vi "Transfer Data to Host DMA.vi"(11 "Settings.DMA":cluster{"# of Injectors":u8}={"# of Injectors"=6}) -> (2 "Intermediate Time Out?":bool, 3 "Host DMA Out?":bool)   [LabVIEW 2015]
uses:
  <vilib>/rvi/DataTransferAndStorage/Container/Common/niFpgaContainerExecOnDevCompGetState.vi
  <vilib>/rvi/Emulation/niFpgaEmulationIsFPGAContextNoSignature.vi
  <vilib>/rvi/Emulation/niFpgaSctlEmulationGetInTimedLoop.vi
  <vilib>/rvi/errors/niFpgaSetErrorForExecOnDevCompSimple.vi
  <vilib>/rvi/eio/common/nirviEmuReportErrorAndStop.vi
  <vilib>/rvi/DataTransferAndStorage/Container/Common/niFpgaContainerGetUniqueNameForEmu.vi
  <vilib>/rvi/FIFO/Fifo_Resource/nirvififoEmulationSetSize.vi
  <vilib>/rvi/FIFO/Fifo_Resource/nirviFifoEmulationQueueMgr.vi
  <instcachedir>/0/nirviFifoEmulationQueueMgr_E5CAEC123FF24DC58D834DCA3CDAA9B5.lvgen/nirviFifoEmulationQueueMgr_E5CAEC123FF24DC58D834DCA3CDAA9B5_001.vi
  <vilib>/rvi/FIFO/Fifo_Resource/nirvififoEmulationDetermineInputValidOut.vi
  <vilib>/rvi/FIFO/Fifo_Resource/nirvififoEmulationCreateLock.vi
  <vilib>/rvi/Emulation/niFpgaProcessEmulError.vi
  <vilib>/rvi/FIFO/Fifo_Resource/nirvififoEmulationObtainLock.vi
  <vilib>/rvi/FIFO/Fifo_Resource/nirvififoEmulationReleaseLock.vi
  <vilib>/rvi/occurrence/nirviWaitOnOccurrenceBase.vi
  <vilib>/rvi/errors/nirviReportUnexpectedCaseInternalError.vi
  <vilib>/rvi/errors/nirviReportUnexpectedCaseInternalError (U32).vi
  <vilib>/Utility/error.llb/Clear Errors.vi
  <vilib>/rvi/interface/RandomDataEmulation/niFpgaRandomDataHandleErrors.vi
  <instcachedir>/0/nirviFifoEmulationQueueMgr_E5CAEC123FF24DC58D834DCA3CDAA9B5.lvgen/nirviFifoEmulationQueueMgr_E5CAEC123FF24DC58D834DCA3CDAA9B5_008.vi
  <vilib>/rvi/DataTransferAndStorage/Container/XNode/niFpgaContainer.xnode
  <vilib>/rvi/FIFO/Fifo_Resource/niFpgaFifoEmulationRefIn.vi
  <vilib>/rvi/interface/RandomDataEmulation/nirviRandomDataFpgaReadWriteTemplate.vi
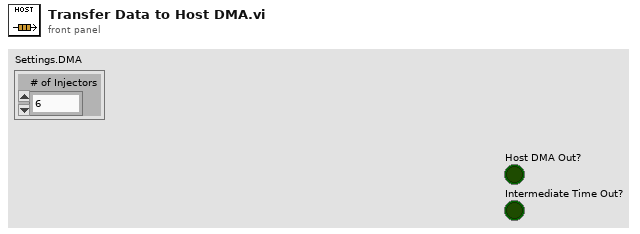
[diagram p1: front panel]
types:
  T1 = cluster{"# of samples captured":u16, "# Transition Elements":u16, "Injector Index":u8, "Iteration":u32}
  T2 = enum8{"Wait on Transfer", "Transfer Injector Index", "Transfer # of Samples", "Transfer # of Transitions", "Transfer Transitions", "Transfer Voltage Samples", "Transfer Current Samples"}
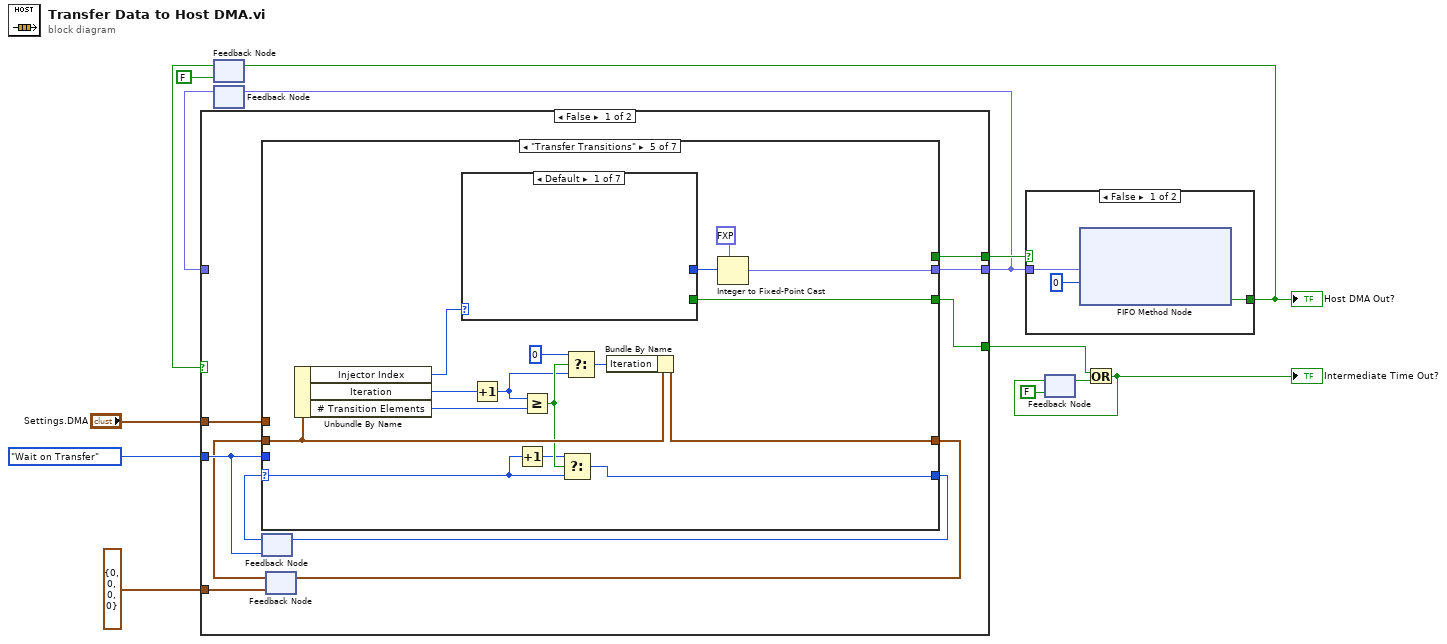
[diagram p0: block diagram]
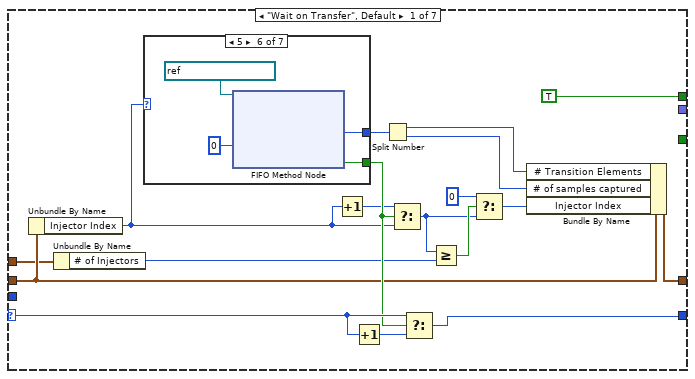
[diagram p2: hidden frame]
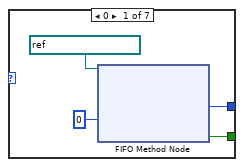
[diagram p3: hidden frame]
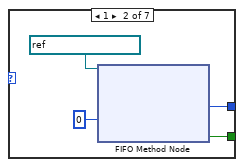
[diagram p4: hidden frame]
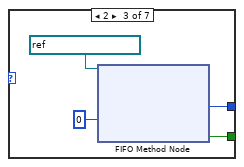
[diagram p5: hidden frame]
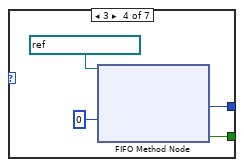
[diagram p6: hidden frame]
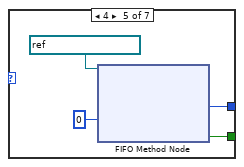
[diagram p7: hidden frame]
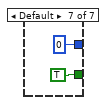
[diagram p8: hidden frame]
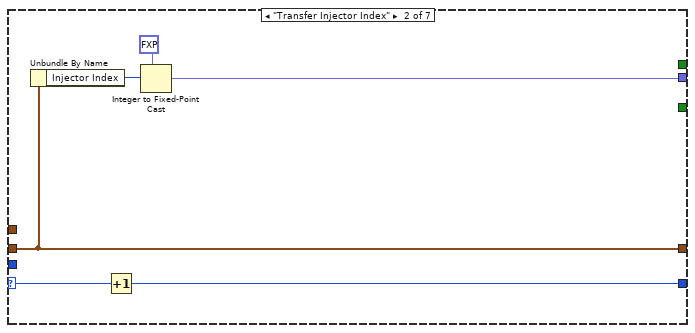
[diagram p9: hidden frame]
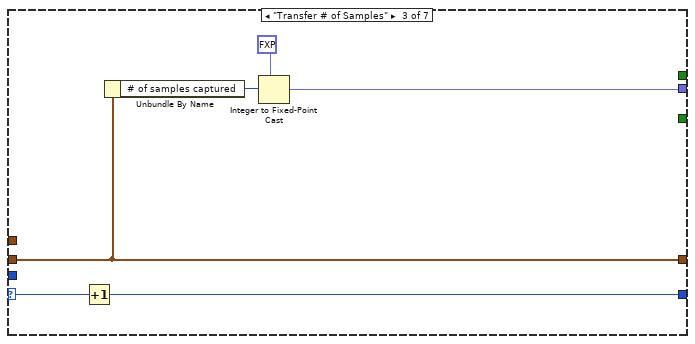
[diagram p10: hidden frame]
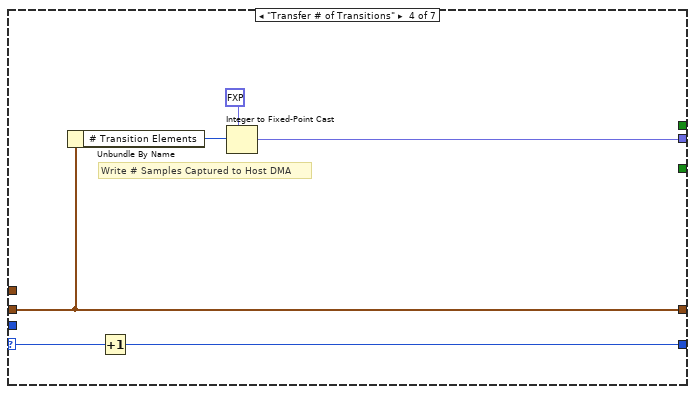
[diagram p11: hidden frame]
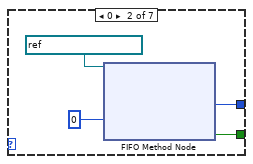
[diagram p12: hidden frame]
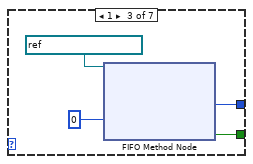
[diagram p13: hidden frame]
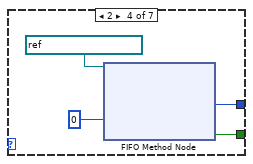
[diagram p14: hidden frame]
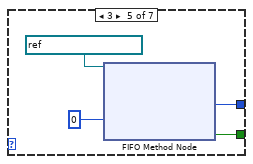
[diagram p15: hidden frame]
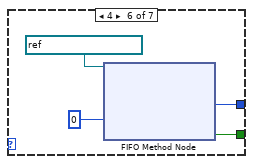
[diagram p16: hidden frame]
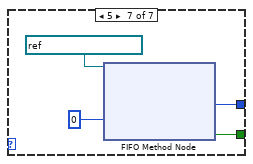
[diagram p17: hidden frame]
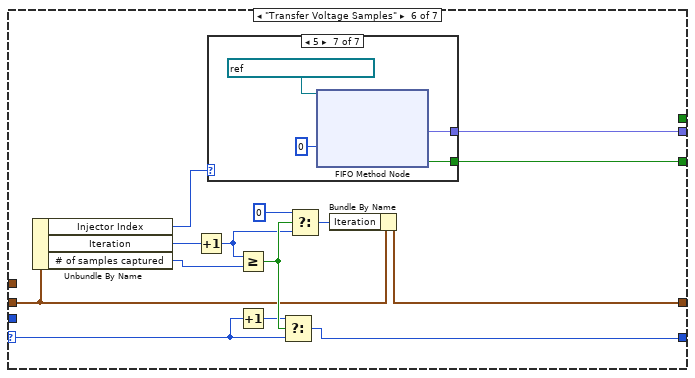
[diagram p18: hidden frame]
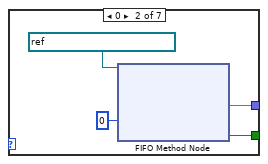
[diagram p20: hidden frame]
diagram:
  n1 = feedback #1(FALSE ("Timed Out?")) -> (w8:bool)
  n2 = feedback #2() -> (w5:fxp<+/-,32,8>)  [unwired: 1 in]
  n3 = case shown="False" w8 {
    tunnel: [w23 w203] -> w6
    tunnel: [w22 w202] -> w10
    tunnel: T2."Wait on Transfer" -> [w19 _]
    tunnel: [w18 w202] -> w1
    tunnel: "Settings.DMA" -> [w17 _]
    tunnel: T1 {"# of samples captured"=0, "# Transition Elements"=0, "Injector Index"=0, "Iteration"=0} ("Local.Data") -> [w14 _]
    tunnel: w5 -> [_ w203]
    frame False {
      n4 = feedback #3(w19) -> (w20:T2)
      n5 = feedback #4(w14) -> (w15:T1)
      n6 = case shown="\"Transfer Transitions\"" w20 {
        selector: w20 -> [w39 w73 w77 w83 w92 w132 w170]
        tunnel: w15 -> [w28 w70 w75 w80 w99 w130 w169]
        tunnel: [w37 w70 w75 w80 w100 w129 w167] -> w16
        tunnel: [w36 w72 w76 w82 w91 w131 w166] -> w21
        tunnel: [_ w69 w74 w81 w87 w128 w177] -> w23
        tunnel: [TRUE _ _ _ _ _ _] -> w22
        tunnel: w19 -> [_ _ _ _ _ _ w165]
        tunnel: [_ _ _ _ w86 w126 w164] -> w18
        tunnel: w17 -> [w25 _ _ _ _ _ _]
        frame "Wait on Transfer", Default {
          n7 = Unbundle By Name(w28) -> ("Injector Index"=w27:u8)
          n8 = Unbundle By Name(w25) -> ("# of Injectors"=w24:u8)
          n9 = case shown="5" w27 {
            tunnel: [w44 w48 w52 w56 w60 w64 u32 0 ("Element")] -> w41
            tunnel: [w43 w47 w51 w55 w59 w63 TRUE ("Timed Out?")] -> w33
            frame 0 {
              n10 = xnode ("FIFO Method Node")("Timeout"=0, "FIFO In"=refnum<k21> "Event Capture 0") -> ("Element"=w44:u32, "Timed Out?"=w43:bool)  [unwired: 1 out]
            }
            frame 1 {
              n11 = xnode ("FIFO Method Node")("Timeout"=0, "FIFO In"=refnum<k21> "Event Capture 1") -> ("Element"=w48:u32, "Timed Out?"=w47:bool)  [unwired: 1 out]
            }
            frame 2 {
              n12 = xnode ("FIFO Method Node")("Timeout"=0, "FIFO In"=refnum<k21> "Event Capture 2") -> ("Element"=w52:u32, "Timed Out?"=w51:bool)  [unwired: 1 out]
            }
            frame 3 {
              n13 = xnode ("FIFO Method Node")("Timeout"=0, "FIFO In"=refnum<k21> "Event Capture 3") -> ("Element"=w56:u32, "Timed Out?"=w55:bool)  [unwired: 1 out]
            }
            frame 4 {
              n14 = xnode ("FIFO Method Node")("Timeout"=0, "FIFO In"=refnum<k21> "Event Capture 4") -> ("Element"=w60:u32, "Timed Out?"=w59:bool)  [unwired: 1 out]
            }
            frame 5 {
              n15 = xnode ("FIFO Method Node")("Timeout"=0, "FIFO In"=refnum<k21> "Event Capture 5") -> ("Element"=w64:u32, "Timed Out?"=w63:bool)  [unwired: 1 out]
            }
            frame Default {
            }
          }
          n16 = Increment(x=w27) -> (x+1=w32:u8)
          n17 = Increment(x=w39) -> (x+1=w40:T2)
          n18 = Split Number(x=w41) -> (hi(x)=w34:u16, lo(x)=w38:u16)
          n19 = Select(t=w32, s=w33, f=w27) -> (s? t:f=w30:u8)
          n20 = Select(t=w39, s=w33, f=w40) -> (s? t:f=w36:T2)
          n21 = Greater Or Equal?(x=w30, y=w24) -> (x >= y?=w31:bool)
          n22 = Select(t=u8 0, s=w31, f=w30) -> (s? t:f=w26:u8)
          n23 = Bundle By Name(cluster=w28, "# Transition Elements"=w34, "# of samples captured"=w38, "Injector Index"=w26) -> (w37:T1)
        }
        frame "Transfer Injector Index" {
          n24 = Unbundle By Name(w70) -> ("Injector Index"=w71:u8)
          n25 = Increment(x=w73) -> (x+1=w72:T2)
          n26 = Integer to Fixed-Point Cast(fixed-point type=fxp<+/-,32,8> 0.0, integer=w71) -> (fixed-point=w69:fxp<+/-,32,8>)
        }
        frame "Transfer # of Samples" {
          n27 = Increment(x=w77) -> (x+1=w76:T2)
          n28 = Unbundle By Name(w75) -> ("# of samples captured"=w78:u16)
          n29 = Integer to Fixed-Point Cast(fixed-point type=fxp<+/-,32,8> 0.0, integer=w78) -> (fixed-point=w74:fxp<+/-,32,8>)
        }
        frame "Transfer # of Transitions" {
          # "Write # Samples Captured to Host DMA"
          n30 = Unbundle By Name(w80) -> ("# Transition Elements"=w84:u16)
          n31 = Increment(x=w83) -> (x+1=w82:T2)
          n32 = Integer to Fixed-Point Cast(fixed-point type=fxp<+/-,32,8> 0.0, integer=w84) -> (fixed-point=w81:fxp<+/-,32,8>)
        }
        frame "Transfer Transitions" {
          n33 = Unbundle By Name(w99) -> ("Injector Index"=w101:u8, "Iteration"=w95:u32, "# Transition Elements"=w96:u16)
          n34 = case shown="Default" w101 {
            tunnel: [_ w105 w109 w113 w117 w121 w125] -> w97
            tunnel: [_ w103 w107 w111 w115 w119 w123] -> w86
            frame Default {
            }
            frame 0 {
              n35 = xnode ("FIFO Method Node")("Timeout"=0, "FIFO In"=refnum<k21> "Transition FIFO 0" ("Transition FIFO")) -> ("Element"=w105:u32, "Timed Out?"=w103:bool)  [unwired: 1 out]
            }
            frame 1 {
              n36 = xnode ("FIFO Method Node")("Timeout"=0, "FIFO In"=refnum<k21> "Transition FIFO 1" ("Transition FIFO")) -> ("Element"=w109:u32, "Timed Out?"=w107:bool)  [unwired: 1 out]
            }
            frame 2 {
              n37 = xnode ("FIFO Method Node")("Timeout"=0, "FIFO In"=refnum<k21> "Transition FIFO 2" ("Transition FIFO")) -> ("Element"=w113:u32, "Timed Out?"=w111:bool)  [unwired: 1 out]
            }
            frame 3 {
              n38 = xnode ("FIFO Method Node")("Timeout"=0, "FIFO In"=refnum<k21> "Transition FIFO 3" ("Transition FIFO")) -> ("Element"=w117:u32, "Timed Out?"=w115:bool)  [unwired: 1 out]
            }
            frame 4 {
              n39 = xnode ("FIFO Method Node")("Timeout"=0, "FIFO In"=refnum<k21> "Transition FIFO 4" ("Transition FIFO")) -> ("Element"=w121:u32, "Timed Out?"=w119:bool)  [unwired: 1 out]
            }
            frame 5 {
              n40 = xnode ("FIFO Method Node")("Timeout"=0, "FIFO In"=refnum<k21> "Transition FIFO 5" ("Transition FIFO")) -> ("Element"=w125:u32, "Timed Out?"=w123:bool)  [unwired: 1 out]
            }
          }
          n41 = Increment(x=w95) -> (x+1=w89:u32)
          n42 = Increment(x=w92) -> (x+1=w93:T2)
          n43 = Greater Or Equal?(x=w89, y=w96) -> (x >= y?=w94:bool)
          n44 = Select(t=w93, s=w94, f=w92) -> (s? t:f=w91:T2)
          n45 = Select(t=u32 0, s=w94, f=w89) -> (s? t:f=w88:u32)
          n46 = Bundle By Name(cluster=w99, "Iteration"=w88) -> (w100:T1)
          n47 = Integer to Fixed-Point Cast(fixed-point type=fxp<+/-,32,8> 0.0, integer=w97) -> (fixed-point=w87:fxp<+/-,32,8>)
        }
        frame "Transfer Voltage Samples" {
          n48 = Unbundle By Name(w130) -> ("Injector Index"=w139:u8, "Iteration"=w133:u32, "# of samples captured"=w127:u16)
          n49 = Increment(x=w133) -> (x+1=w135:u32)
          n50 = case shown="5" w139 {
            tunnel: [_ w142 w146 w150 w154 w158 w162] -> w128
            tunnel: [_ w141 w145 w149 w153 w157 w161] -> w126
            frame Default {
            }
            frame 0 {
              n51 = xnode ("FIFO Method Node")("Timeout"=0, "FIFO In"=refnum<k21> "Intermediate Voltage 0" ("Voltage FIFO")) -> ("Element"=w142:fxp<+/-,32,8>, "Timed Out?"=w141:bool)  [unwired: 1 out]
            }
            frame 1 {
              n52 = xnode ("FIFO Method Node")("Timeout"=0, "FIFO In"=refnum<k21> "Intermediate Voltage 1" ("Voltage FIFO")) -> ("Element"=w146:fxp<+/-,32,8>, "Timed Out?"=w145:bool)  [unwired: 1 out]
            }
            frame 2 {
              n53 = xnode ("FIFO Method Node")("Timeout"=0, "FIFO In"=refnum<k21> "Intermediate Voltage 2" ("Voltage FIFO")) -> ("Element"=w150:fxp<+/-,32,8>, "Timed Out?"=w149:bool)  [unwired: 1 out]
            }
            frame 3 {
              n54 = xnode ("FIFO Method Node")("Timeout"=0, "FIFO In"=refnum<k21> "Intermediate Voltage 3" ("Voltage FIFO")) -> ("Element"=w154:fxp<+/-,32,8>, "Timed Out?"=w153:bool)  [unwired: 1 out]
            }
            frame 4 {
              n55 = xnode ("FIFO Method Node")("Timeout"=0, "FIFO In"=refnum<k21> "Intermediate Voltage 4" ("Voltage FIFO")) -> ("Element"=w158:fxp<+/-,32,8>, "Timed Out?"=w157:bool)  [unwired: 1 out]
            }
            frame 5 {
              n56 = xnode ("FIFO Method Node")("Timeout"=0, "FIFO In"=refnum<k21> "Intermediate Voltage 5" ("Voltage FIFO")) -> ("Element"=w162:fxp<+/-,32,8>, "Timed Out?"=w161:bool)  [unwired: 1 out]
            }
          }
          n57 = Greater Or Equal?(x=w135, y=w127) -> (x >= y?=w138:bool)
          n58 = Increment(x=w132) -> (x+1=w137:T2)
          n59 = Select(t=w137, s=w138, f=w132) -> (s? t:f=w131:T2)
          n60 = Select(t=u32 0, s=w138, f=w135) -> (s? t:f=w134:u32)
          n61 = Bundle By Name(cluster=w130, "Iteration"=w134) -> (w129:T1)
        }
        frame "Transfer Current Samples" {
          n62 = Unbundle By Name(w169) -> ("Injector Index"=w168:u8, "Iteration"=w172:u32, "# of samples captured"=w171:u16)
          n63 = Increment(x=w172) -> (x+1=w174:u32)
          n64 = case shown="0" w168 {
            tunnel: [_ w180 w184 w188 w192 w196 w200] -> w177
            tunnel: [_ w179 w183 w187 w191 w195 w199] -> w164
            frame Default {
            }
            frame 0 {
              n65 = xnode ("FIFO Method Node")("Timeout"=0, "FIFO In"=refnum<k21> "Intermediate Current 0") -> ("Element"=w180:fxp<+/-,32,8>, "Timed Out?"=w179:bool)  [unwired: 1 out]
            }
            frame 1 {
              n66 = xnode ("FIFO Method Node")("Timeout"=0, "FIFO In"=refnum<k21> "Intermediate Current 1") -> ("Element"=w184:fxp<+/-,32,8>, "Timed Out?"=w183:bool)  [unwired: 1 out]
            }
            frame 2 {
              n67 = xnode ("FIFO Method Node")("Timeout"=0, "FIFO In"=refnum<k21> "Intermediate Current 2") -> ("Element"=w188:fxp<+/-,32,8>, "Timed Out?"=w187:bool)  [unwired: 1 out]
            }
            frame 3 {
              n68 = xnode ("FIFO Method Node")("Timeout"=0, "FIFO In"=refnum<k21> "Intermediate Current 3") -> ("Element"=w192:fxp<+/-,32,8>, "Timed Out?"=w191:bool)  [unwired: 1 out]
            }
            frame 4 {
              n69 = xnode ("FIFO Method Node")("Timeout"=0, "FIFO In"=refnum<k21> "Intermediate Current 4") -> ("Element"=w196:fxp<+/-,32,8>, "Timed Out?"=w195:bool)  [unwired: 1 out]
            }
            frame 5 {
              n70 = xnode ("FIFO Method Node")("Timeout"=0, "FIFO In"=refnum<k21> "Intermediate Current 5") -> ("Element"=w200:fxp<+/-,32,8>, "Timed Out?"=w199:bool)  [unwired: 1 out]
            }
          }
          n71 = Greater Or Equal?(x=w174, y=w171) -> (x >= y?=w176:bool)
          n72 = Select(t=u32 0, s=w176, f=w174) -> (s? t:f=w173:u32)
          n73 = Select(t=w165, s=w176, f=w170) -> (s? t:f=w166:T2)
          n74 = Bundle By Name(cluster=w169, "Iteration"=w173) -> (w167:T1)
        }
      }
      n75 = feedback-in #3(w21) -> ()
      n76 = feedback-in #4(w16) -> ()
    }
    frame True {
      w202 = FALSE
    }
  }
  n77 = feedback-in #2(w6) -> ()
  n78 = case shown="False" w10 {
    tunnel: w6 -> [w205 _]
    tunnel: [w204 FALSE ("Timed Out?")] -> w9
    frame False {
      n79 = xnode ("FIFO Method Node")("Element"=w205, "Timeout"=0) -> ("Timed Out?"=w204:bool)  [unwired: 1 in, 1 out]
    }
    frame True {
    }
  }
  "Host DMA Out?" <- w9
  n80 = feedback-in #1(w9) -> ()
  n81 = feedback #5(FALSE ("Timed Out?")) -> (w3:bool)
  n82 = Or(x=w1, y=w3) -> (x .or. y?=w2:bool)
  "Intermediate Time Out?" <- w2
  n83 = feedback-in #5(w2) -> ()
